vi "OpenAndRunVi (SubVI) — with saw.vi"(11 "VI in":refnum<vi>) -> ()   [LabVIEW 2017]
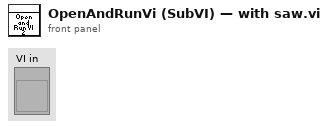
[diagram p1: front panel]
types:
  T1 = enum32{"Invalid", "Standard", "Closed", "Hidden", "Minimized", "Maximized"}
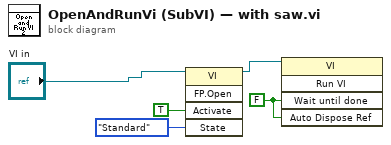
[diagram p0: block diagram]
diagram:
  w5 = FALSE ("Wait Until Done")
  n1 = invoke class="VI" method="FP.Open"(reference="VI in", "Activate"=TRUE ("Activate?"), "State"=T1."Standard") -> (reference out=w4:refnum<vi>)  [unwired: 2 in, 4 out]
  n2 = invoke class="VI" method="Run VI"(reference=w4, "Wait until done"=w5, "Auto Dispose Ref"=w5) -> ()  [unwired: 2 in, 5 out]
